vi "一维数组移位函数.vi"() -> ()   [LabVIEW 2014]
panel:
  in  "停止":bool
  out "循环左移":bool[](array[boolean])
  out "循环右移":bool[](array[boolean])
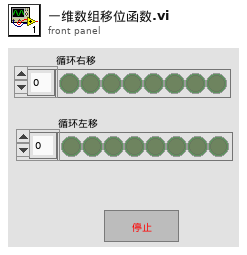
[diagram p1: front panel]
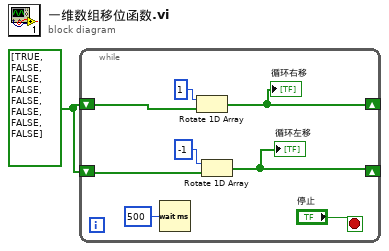
[diagram p0: block diagram]
diagram:
  w1 = bool[] [TRUE, FALSE, FALSE, FALSE, FALSE, FALSE, FALSE, FALSE]
  n1 = while {
    shift-right: [w8] -> _
    shift-left: w1 -> [w9]
    shift-right: [w5] -> _
    shift-left: w1 -> [w6]
    stop <- "停止" stop-if-true
    n2 = Wait (ms)(milliseconds to wait=u32 500 ("等待时间（毫秒）")) -> ()  [unwired: 1 out]
    n3 = Rotate 1D Array(1:w9, 2:1 ("n")) -> (0:w8:bool[])
    "循环右移" <- w8
    n4 = Rotate 1D Array(1:w6, 2:-1 ("n")) -> (0:w5:bool[])
    "循环左移" <- w5
  }
